vi "CTRE_PigeonIMU_GetStatusString.vi"(8 "error in (no error)":errorcluster, 11 "PigeonIMUDevRef":T1={"DeviceStatus"={"status"=FALSE, "code"=0, "source"=""}, "Device Number"=0, "Type"=352321536, "Device ID"=0} {"Type" items=["CAN"=352321536, "TalonSRX"=33554432]}) -> (0 "error out":errorcluster, 2 "Pigeon Status":string, 3 "PigeonIMUDevRef":T1={"DeviceStatus"={"status"=FALSE, "code"=0, "source"=""}, "Device Number"=0, "Type"=352321536, "Device ID"=0} {"Type" items=["CAN"=352321536, "TalonSRX"=33554432]})   [LabVIEW 2016]
doc: "Generates a String that describes the current status of the Pigeon. Usually used for feedback of the calibration process."
uses:
  <vilib>/Rock Robotics/WPI/ThirdParty/Sensors/Pigeon IMU/CTRE_PigeonIMU_DeviceRef.ctl
  <vilib>/Rock Robotics/WPI/ThirdParty/Sensors/Pigeon IMU/CTRE_PigeonIMU_ConnectionType.ctl
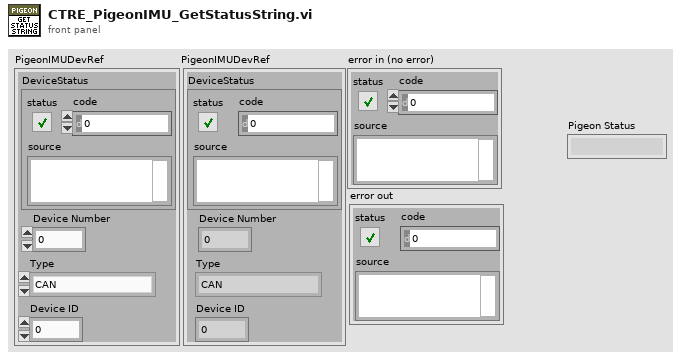
[diagram p1: front panel]
types:
  T1 = typedef "CTRE_PigeonIMU_DeviceRef.ctl" = cluster{"DeviceStatus":errorcluster, "Device Number":u8, "Type":T2, "Device ID":u32}
  T2 = typedef "CTRE_PigeonIMU_ConnectionType.ctl" = u32
  T3 = typedef "CTRE_PigeonIMU_GlobalStatus.ctl" = cluster{"PigeonState":T4, "FusedHeading":cluster{"Heading":dbl, "Valid?":bool, "Fusing?":bool}, "YPR":cluster{"Yaw":dbl, "Pitch":dbl, "Roll":dbl}, "Compass":cluster{"Heading":dbl, "Magnitude":dbl, "Absolute Heading":dbl}, "Accelerometer":cluster{"Biased":cluster{"X":i16, "Y":i16, "Z":i16, "Norm":i16}, "Angles":cluster{"XZ Tilt":dbl, "YZ Tilt":dbl, "XY Tilt":dbl}}, "Magnetometer":cluster{"Raw":cluster{"X":i16, "Y":i16, "Z":i16}, "Biased":cluster{"X":i16, "Y":i16, "Z":i16}}, "Gyro":cluster{"X":dbl, "Y":dbl, "Z":dbl, "Norm":dbl}, "6D Quaternian":cluster{"W":dbl, "X":dbl, "Y":dbl, "Z":dbl}, "Temp. (C)":dbl, "UpTime":u32, "StartupStatus":cluster{"ResetCount":i32, "ResetFlags":i32, "FirmwareVersion":i32, "HasReset?":bool}, "Calibration":cluster{"CurrentMode":T5, "LastCalError":i32, "CalBooting?":bool}, "CAN Error":errorcluster, "AccumGyro":cluster{"X":dbl, "Y":dbl, "Z":dbl}}
  T4 = typedef "CTRE_PigeonIMU_PigeonState.ctl" = enum16{"NoComm", "Initializing", "Ready", "UserCalibration"}
  T5 = typedef "CTRE_PigeonIMU_CalibrationMode.ctl" = u16
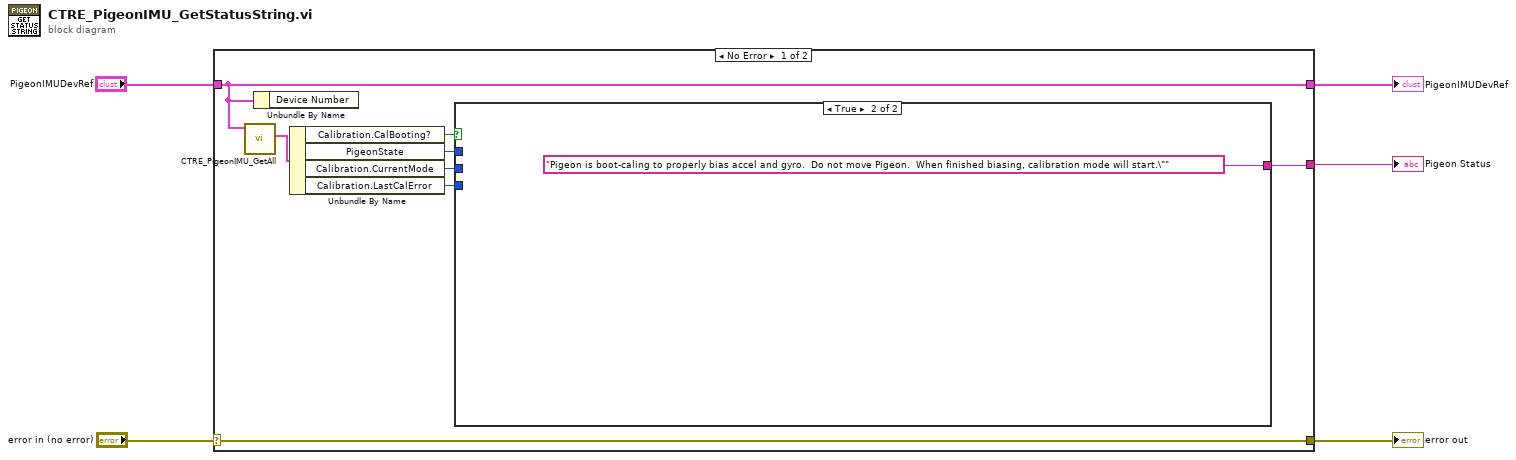
[diagram p0: block diagram]
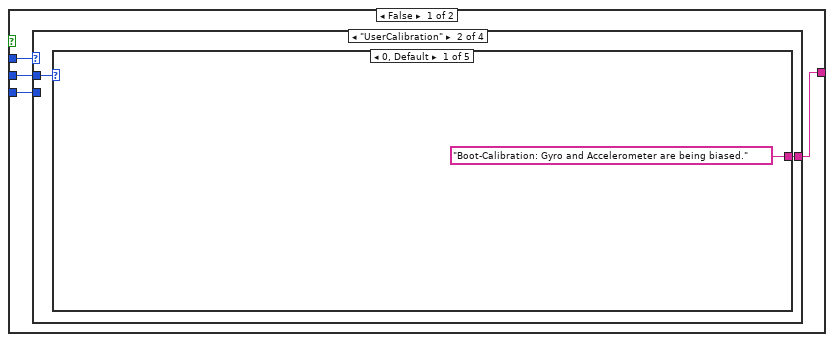
[diagram p2: hidden frame]
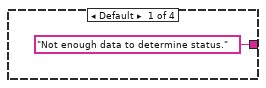
[diagram p3: hidden frame]
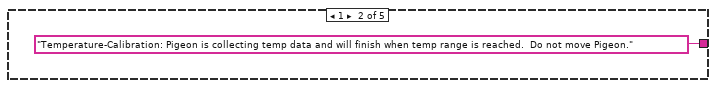
[diagram p4: hidden frame]
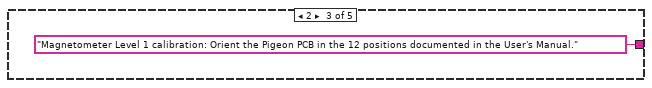
[diagram p5: hidden frame]
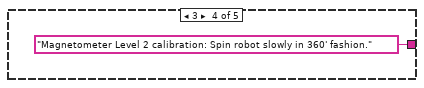
[diagram p6: hidden frame]
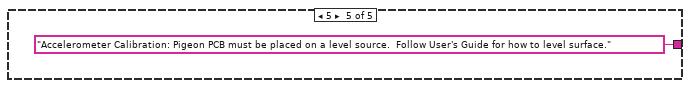
[diagram p7: hidden frame]
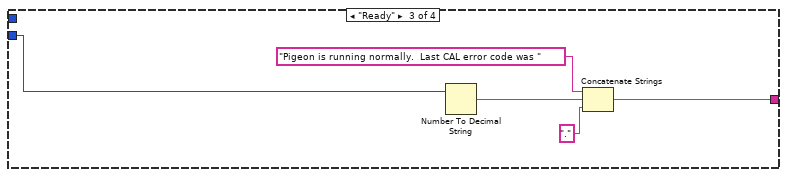
[diagram p8: hidden frame]
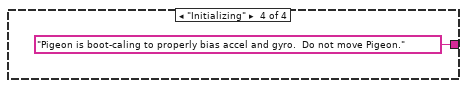
[diagram p9: hidden frame]
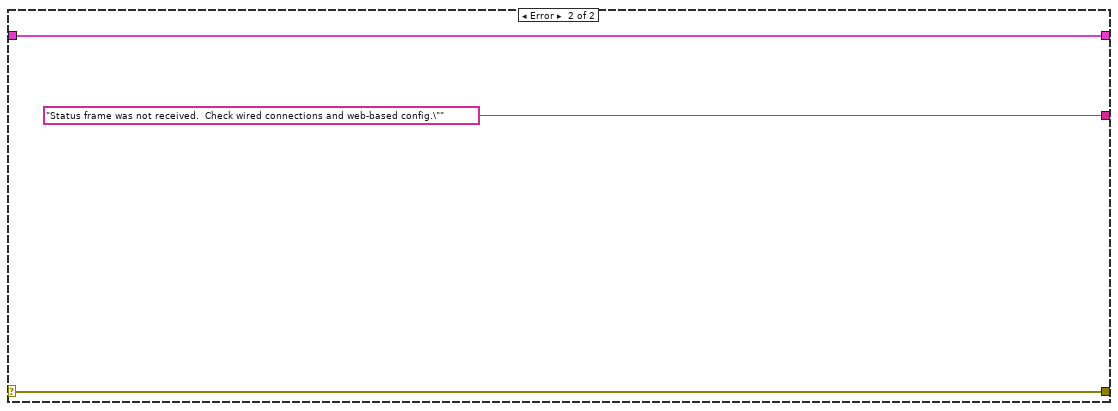
[diagram p10: hidden frame]
diagram:
  n1 = case shown="No Error" "error in (no error)" {
    selector: "error in (no error)" -> [w13 w33]
    tunnel: [w13 w33] -> w4
    tunnel: [w12 w35] -> w2
    tunnel: "PigeonIMUDevRef" -> [w12 w35]
    tunnel: [w9 "Status frame was not received.  Check wired connections and web-based config.\""] -> w1
    frame No Error {
      n2 = call <vilib>:"CTRE_PigeonIMU_GetAll.vi"("PigeonIMUDevRef"=w12) -> ("Get All"=w11:T3)  [unwired: 8 in, 2 out]
      n3 = Unbundle By Name(w12) -> ()  [unwired: 1 out]
      n4 = Unbundle By Name(w11) -> ("Calibration.CalBooting?"=w10:bool, "PigeonState"=w8:T4, "Calibration.CurrentMode"=w7:T5, "Calibration.LastCalError"=w6:i32)
      n5 = case shown="True" w10 {
        tunnel: [w15 "Pigeon is boot-caling to properly bias accel and gyro.  Do not move Pigeon.  When finished biasing, calibration mode will start.\""] -> w9
        tunnel: w8 -> [w17 _]
        tunnel: w7 -> [w16 _]
        tunnel: w6 -> [w14 _]
        frame False {
          n6 = case shown="\"UserCalibration\"" w17 {
            tunnel: w16 -> [_ w20 _ _]
            tunnel: ["Not enough data to determine status." w19 w30 "Pigeon is boot-caling to properly bias accel and gyro.  Do not move Pigeon."] -> w15
            tunnel: w14 -> [_ _ w26 _]
            frame Default {
            }
            frame "UserCalibration" {
              n7 = case shown="0, Default" w20 {
                tunnel: ["Boot-Calibration: Gyro and Accelerometer are being biased." "Temperature-Calibration: Pigeon is collecting temp data and will finish when temp range is reached.  Do not move Pigeon." "Magnetometer Level 1 calibration: Orient the Pigeon PCB in the 12 positions documented in the User's Manual." "Magnetometer Level 2 calibration: Spin robot slowly in 360' fashion." "Accelerometer Calibration: Pigeon PCB must be placed on a level source.  Follow User's Guide for how to level surface."] -> w19
                frame 0, Default {
                }
                frame 1 {
                }
                frame 2 {
                }
                frame 3 {
                }
                frame 5 {
                }
              }
            }
            frame "Ready" {
              n8 = Number To Decimal String(number=w26) -> (decimal integer string=w27:string)  [unwired: 1 in]
              n9 = Concatenate Strings("Pigeon is running normally.  Last CAL error code was " ("string"), w27, "." ("string")) -> (w30:string)
            }
            frame "Initializing" {
            }
          }
        }
        frame True {
        }
      }
    }
    frame Error {
    }
  }
  "PigeonIMUDevRef" <- w2
  "error out" <- w4
  "Pigeon Status" <- w1
